vi "Fetch Waveforms for One Record with Scope Info Map.vi"(8 "error in (no error)":errorcluster, 9 "fetch record number":i32, 10 "scope info map":T3(c390), 11 "Scope handles":refnum<k15>[](array[refnum])) -> (0 "error out":errorcluster, 1 "waverforms":waveform(dbl)[](array[waveform]), 2 "sites":i32[](array[numeric]), 3 "pins":string[](array[string]))   [LabVIEW 2021, in "PMIC Common.lvlib"]
uses:
  PMIC Common.lvlib
  <instrlib>/niScope/Controls/niScope timestamp type.ctl
  <instrlib>/niScope/Acquire/Fetch/niScope Multi Fetch WDT.vi
  <instrlib>/niScope/Controls/niScope vertical coupling.ctl
  Scope Parameters.ctl
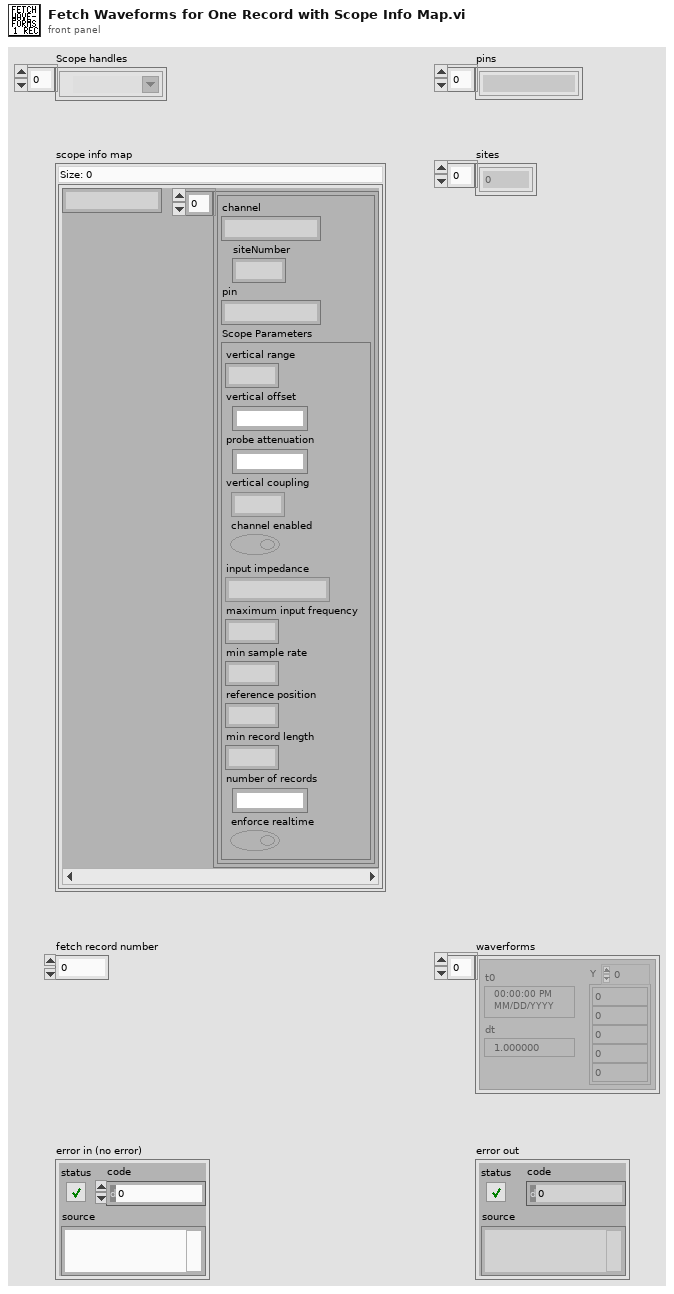
[diagram p1: front panel]
types:
  T1 = typedef "PMIC Common.lvlib/Scope Parameters.ctl" = cluster{"vertical range":dbl, "vertical offset":dbl, "probe attenuation":dbl, "vertical coupling":T2, "channel enabled":bool, "input impedance":u32, "maximum input frequency":dbl, "min sample rate":dbl, "reference position":dbl, "min record length":i32, "number of records":i32, "enforce realtime":bool}
  T2 = typedef "niScope vertical coupling.ctl" = i32
  T3 = map{string, cluster{"channel":string, "siteNumber":i32, "pin":string, "Scope Parameters":T1}[]}
  T4 = cluster{"channel":string, "siteNumber":i32, "pin":string, "Scope Parameters":T1}[]
  T5 = typedef "niScope timestamp type.ctl" = i32
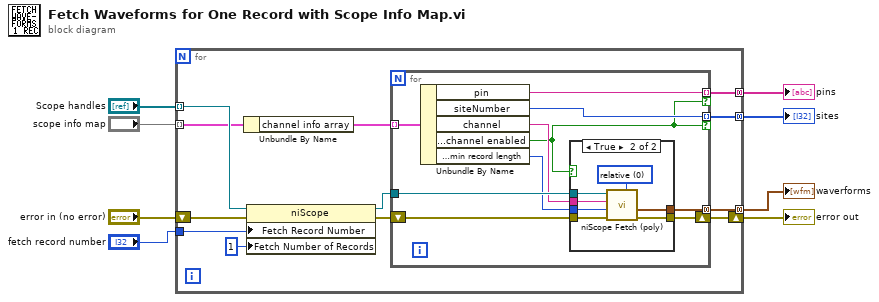
[diagram p0: block diagram]
diagram:
  n1 = for {
    tunnel: "Scope handles" -> [w14] mode=indexing
    shift-right: [w17] -> w4
    shift-left: "error in (no error)" -> [w15]
    tunnel: [w16] -> w3 mode=concatenating
    tunnel: "fetch record number" -> [w13]
    tunnel: "scope info map" -> [w11] mode=indexing
    tunnel: [w10] -> w7 mode=concatenating
    tunnel: [w9] -> w8 mode=concatenating
    n2 = Unbundle By Name(w11) -> ("channel info array"=w12:T4)
    n3 = property class="niScope"(reference=w14, error in=w15, "Fetch Record Number"=w13, "Fetch Number of Records"=1 ("Fetch:Fetch Number of Records")) -> (reference out=w18:refnum<k15>, error out=w19:errorcluster)
    n4 = for {
      tunnel: w18 -> [w29]
      tunnel: [w27] -> w16 mode=concatenating
      shift-right: [w28] -> w17
      shift-left: w19 -> [w30]
      tunnel: w12 -> [w26] mode=indexing
      tunnel: [w24] -> w9 mode=indexing if=w21
      tunnel: [w23] -> w10 mode=indexing if=w21
      n5 = Unbundle By Name(w26) -> ("pin"=w23:string, "siteNumber"=w24:i32, "channel"=w25:string, "Scope Parameters.channel enabled"=w21:bool, "Scope Parameters.min record length"=w22:i32)
      n6 = case shown="True" w21 {
        tunnel: w30 -> [w31 w38]
        tunnel: w29 -> [_ w37]
        tunnel: [w31 w36] -> w28
        tunnel: [_ w35] -> w27
        tunnel: w25 -> [_ w34]
        tunnel: w22 -> [_ w33]
        frame False {
        }
        frame True {
          w32 = T5 0 items=["relative", "absolute"] ("timestamp Type")
          n7 = call-poly <instrlib>:"niScope Fetch (poly).vi"("timestamp Type"=w32, "error in"=w38, "numSamples"=w33, "channels"=w34, "instrument handle"=w37) -> ("error out"=w36:errorcluster, "wfm"=w35:waveform(dbl)[])  [unwired: 3 in, 2 out]
        }
      }
    }
  }
  "sites" <- w8
  "pins" <- w7
  "error out" <- w4
  "waverforms" <- w3
